vi "Template VI.vi"(8 "error in (no error)":errorcluster) -> (0 "error out":errorcluster)   [LabVIEW 2013]
doc: "Statnett PMU Reference Library Template VI with open block diagram\nUse this when creating new VIs in your application"
panel:
  # "INPUT"
  # "INTERMEDIATE"
  # "OUTPUT"
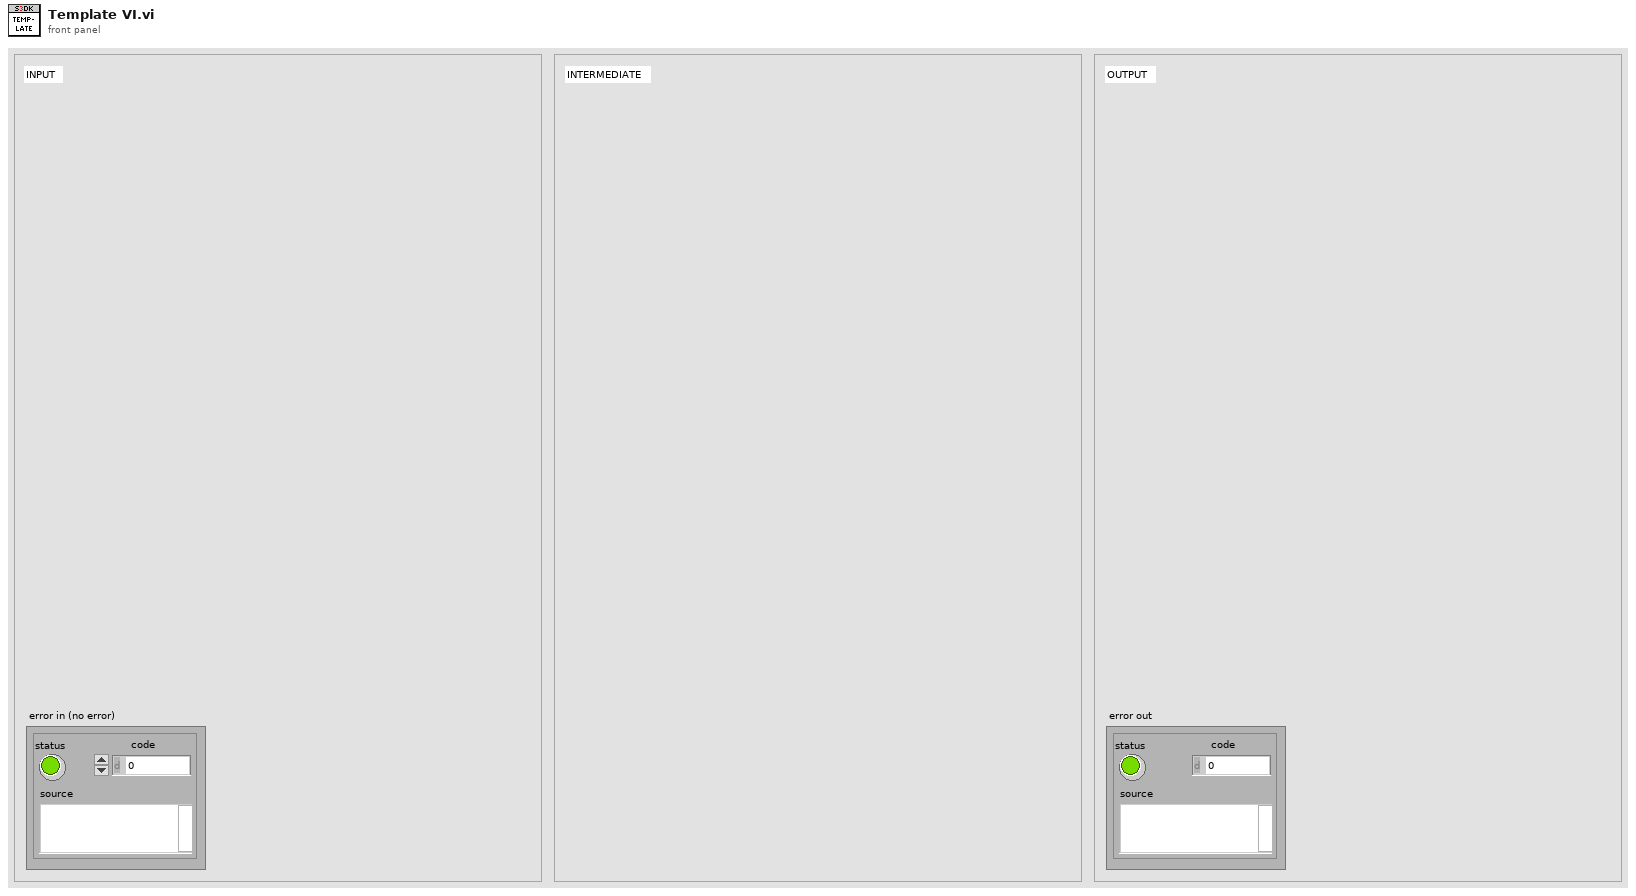
[diagram p1: front panel]
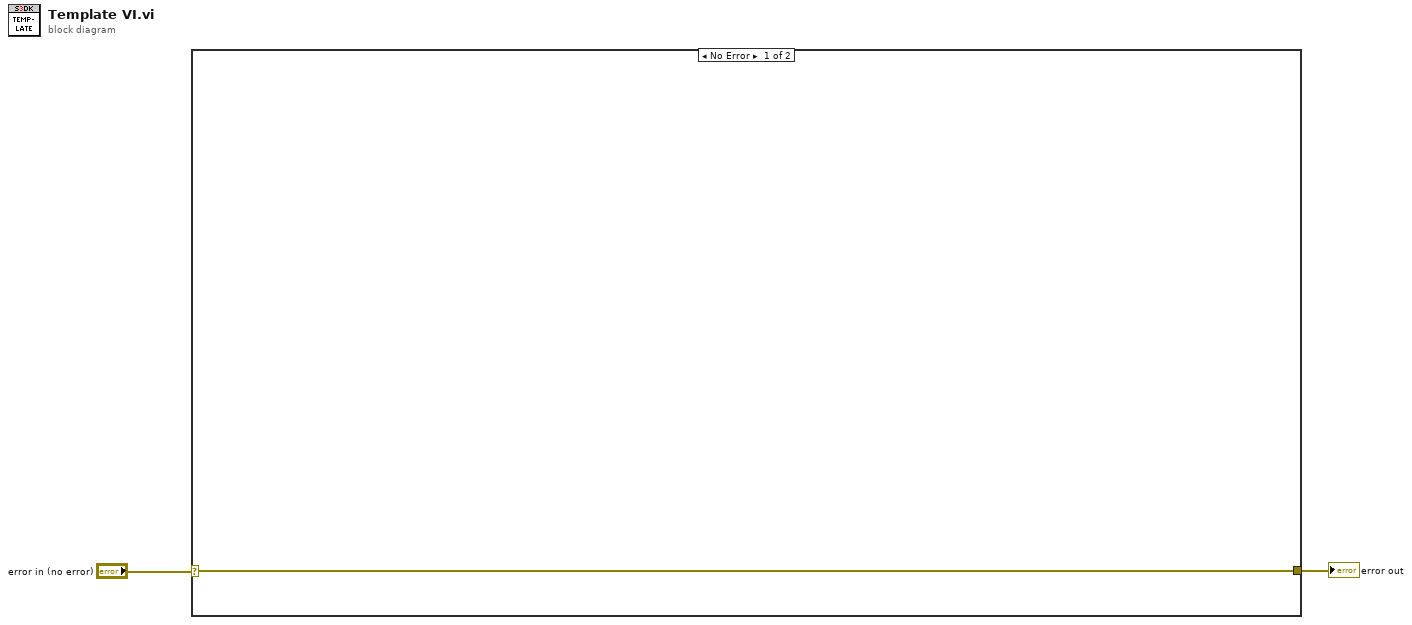
[diagram p0: block diagram]
diagram:
  n1 = case shown="No Error" "error in (no error)" {
    selector: "error in (no error)" -> [w3 w4]
    tunnel: [w3 w4] -> w1
    frame No Error {
    }
    frame Error {
    }
  }
  "error out" <- w1
